vi "Read Command String.vi"(8 "error in (no error)":errorcluster, 11 "RxTxCamera in":refnum<class "RxTxCamera.lvclass">) -> (0 "error out":errorcluster, 2 "String Command":string, 3 "RxTxCamera out":refnum<class "RxTxCamera.lvclass">)   [LabVIEW 2018, in "RxTxCamera.lvclass"]
doc: "Este VI realiza a leitura do tipo de dado que está chegando: comando, header, configuração ou status."
uses:
  RxTxCamera.lvclass
  C:/Users/Cliente/Desktop/Software Echarpe/RxTx/RxTx.lvclass
  RxTx/RxTx.lvclass/RxTx.ctl
  RxTx/RxTx.lvclass
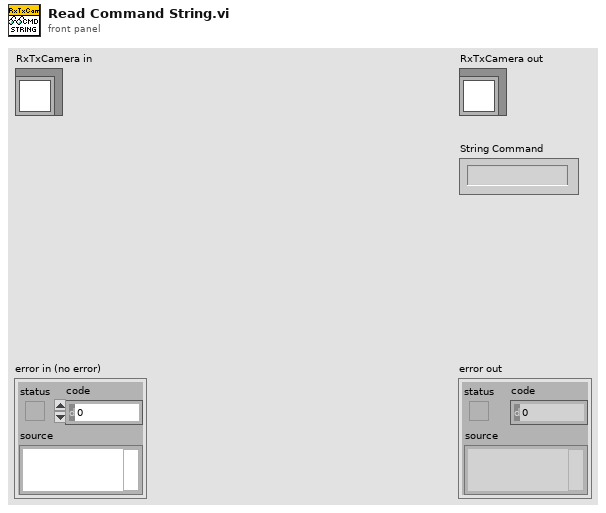
[diagram p1: front panel]
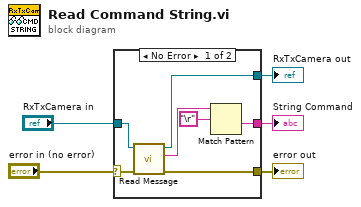
[diagram p0: block diagram]
diagram:
  n1 = case shown="No Error" "error in (no error)" {
    selector: "error in (no error)" -> [w12 w13]
    tunnel: [w11 w13] -> w4
    tunnel: [w9 w14] -> w2
    tunnel: "RxTxCamera in" -> [w10 w14]
    tunnel: [w6 _] -> w1
    frame No Error {
      n2 = call "Read Message.vi"("error in (no error)"=w12, "RxTx in"=w10) -> ("error out"=w11:errorcluster, "Message"=w7:string, "RxTx out"=w9:refnum<class "RxTxCamera.lvclass">)  [unwired: 7 in]
      n3 = Match Pattern(string=w7, regular expression="\r") -> (after substring=w6:string)  [unwired: 1 in, 3 out]
    }
    frame Error {
    }
  }
  "error out" <- w4
  "RxTxCamera out" <- w2
  "String Command" <- w1
